vi "Log File Results.vi"(6 "Media version":string, 7 "Error":string, 8 "error in":errorcluster, 9 "Pass?":string, 10 "OS build":string, 11 "Part Number":string) -> (0 "error out":errorcluster, 3 "File Name":string)   [LabVIEW 2021]
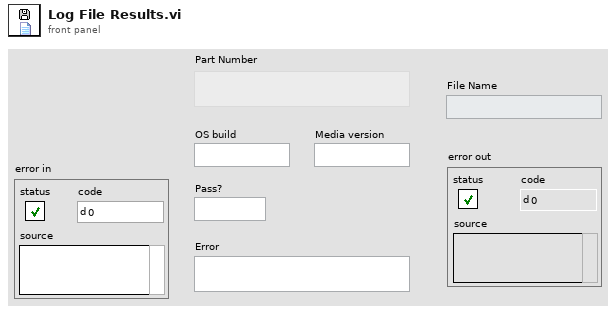
[diagram p1: front panel]
types:
  T1 = enum16{"open", "replace", "create", "open or create", "replace or create", "replace or create with confirmation"}
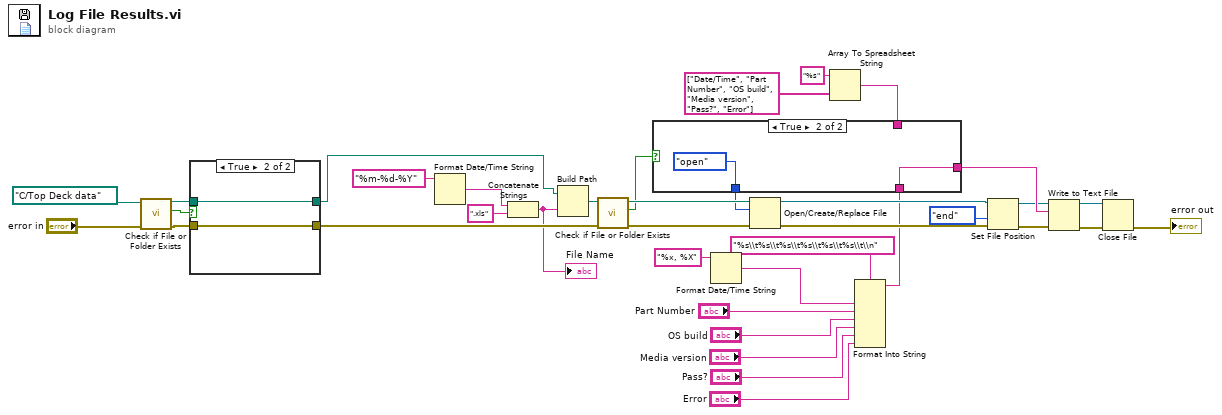
[diagram p0: block diagram]
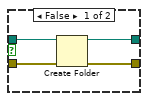
[diagram p2: hidden frame]
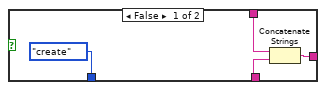
[diagram p3: hidden frame]
diagram:
  n1 = call <vilib>:"Check if File or Folder Exists.vi"("error in (no error)"="error in", "path"=path "C:/Top Deck data") -> ("error out"=w8:errorcluster, "file or folder exists?"=w10:bool, "dup path"=w9:path)  [unwired: 7 in]
  n2 = case shown="True" w10 {
    tunnel: w9 -> [w41 w43]
    tunnel: w8 -> [w40 w42]
    tunnel: [w39 w43] -> w6
    tunnel: [w38 w42] -> w7
    frame False {
      n3 = Create Folder(path (use dialog)=w41, error in=w40) -> (created path=w39:path, error out=w38:errorcluster)  [unwired: 1 in, 1 out]
    }
    frame True {
    }
  }
  n4 = Format Date/Time String(time format string (%c)="%m-%d-%Y") -> (date/time string=w13:string)  [unwired: 2 in]
  n5 = Concatenate Strings(w13, ".xls" ("time format string (%c)")) -> (w1:string)
  "File Name" <- w1
  n6 = Build Path(base path=w6, name or relative path=w1) -> (appended path=w19:path)
  n7 = call <vilib>:"Check if File or Folder Exists.vi"("error in (no error)"=w7, "path"=w19) -> ("error out"=w27:errorcluster, "file or folder exists?"=w23:bool, "dup path"=w26:path)  [unwired: 7 in]
  n8 = Format Date/Time String(time format string (%c)="%x, %X") -> (date/time string=w16:string)  [unwired: 2 in]
  n9 = Array To Spreadsheet String(array=string[] ["Date/Time", "Part Number", "OS build", "Media version", "Pass?", "Error"], 3:"%s" ("format string")) -> (spreadsheet string=w34:string)  [unwired: 1 in]
  n10 = Format Into String(format string="%s\\t%s\\t%s\\t%s\\t%s\\t%s\\t\\n", w16, "Part Number", "OS build", "Media version", "Pass?", "Error") -> (resulting string=w20:string)  [unwired: 2 in, 1 out]
  n11 = case shown="True" w23 {
    tunnel: w34 -> [w47 _]
    tunnel: [w46 w48] -> w33
    tunnel: [T1."create" ("operation (0:open)") T1."open" ("operation (0:open)")] -> w22
    tunnel: w20 -> [w44 w48]
    frame False {
      n12 = Concatenate Strings(w47, w44) -> (w46:string)
    }
    frame True {
    }
  }
  n13 = Open/Create/Replace File(file path (use dialog)=w26, error in=w27, operation (0:open)=w22) -> (refnum out=w25:refnum<file>, error out=w24:errorcluster)  [unwired: 3 in, 1 out]
  n14 = Set File Position(refnum=w25, from (0:start)=enum16{"start", "end", "current"}."end", error in=w24) -> (refnum out=w30:refnum<file>, error out=w29:errorcluster)  [unwired: 1 in]
  n15 = Write to Text File(file (use dialog)=w30, text=w33, error in=w29) -> (refnum out=w31:refnum<file>, error out=w32:errorcluster)  [unwired: 1 in, 1 out]
  n16 = Close File(refnum=w31, error in=w32) -> (error out=→"error out":errorcluster)  [unwired: 1 out]
